vi "TxPkt - Export Channel Configuration.vi"(8 "error in (no error)":errorcluster, 11 "Packet Ref in":T1 format="%.0x") -> (0 "error out":errorcluster, 3 "Packet Ref out":T1 format="%.0x")   [LabVIEW 2019, in "UDP-Custom-Device System Explorer.lvlib"]
uses:
  UDP-Custom-Device System Explorer.lvlib
  <vilib>/NI VeriStand/Custom Device API/Custom Device Item Ref.ctl
  Types/Channel Configuration/Channel Config File Data.ctl
  Property Accessors/Tx Packet Accessors.lvlib
  Property Accessors/Shared Packet Accessors.lvlib
  <vilib>/NI VeriStand/Custom Device API/Custom Device API.lvlib
  Shared/UDP-Custom-Device Shared.lvlib
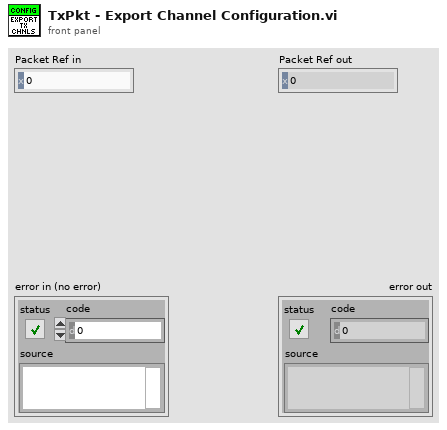
[diagram p1: front panel]
types:
  T1 = typedef "Custom Device API.lvlib/Custom Device Item Ref.ctl" = u64
  T2 = typedef "UDP-Custom-Device System Explorer.lvlib/Channel Config File Data.ctl" = cluster{"Signal Names":string[], "Channel Names":string[], "Channel Data Types":string[], "Channel Descriptions":string[]}
  T3 = typedef "UDP-Custom-Device Shared.lvlib/Shared - Channel Data Type.ctl" = enum16{"Boolean", "Single", "Double", "I8", "I16", "I32", "I64", "U8", "U16", "U32", "U64"}
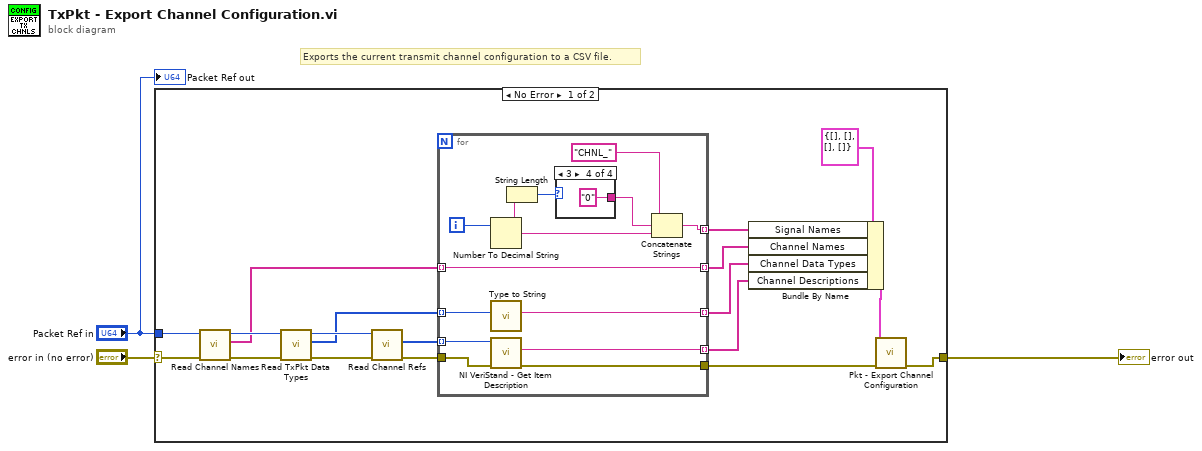
[diagram p0: block diagram]
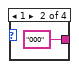
[diagram p3: hidden frame]
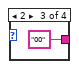
[diagram p4: hidden frame]
diagram:
  # "Exports the current transmit channel configuration to a CSV file."
  n1 = case shown="No Error" "error in (no error)" {
    selector: "error in (no error)" -> [w20 w38]
    tunnel: "Packet Ref in" -> [w21 _]
    tunnel: [w10 w38] -> w2
    frame No Error {
      n2 = call "Read Channel Names.vi"("error in (no error)"=w20, "Node Ptr"=w21) -> ("error out"=w18:errorcluster, "Channel Names"=w12:string[], "Node Ptr out"=w19:T1)  [unwired: 7 in]
      n3 = call "Read TxPkt Data Types.vi"("error in (no error)"=w18, "Node Ptr"=w19) -> ("error out"=w16:errorcluster, "Data types"=w13:T3[], "Node Ptr out"=w17:T1)  [unwired: 7 in]
      n4 = call "Read Channel Refs.vi"("error in (no error)"=w16, "Node Ptr"=w17) -> ("error out"=w15:errorcluster, "Dependent Node Refs"=w14:T1[])  [unwired: 7 in, 1 out]
      n5 = for {
        tunnel: w15 -> [w33]
        tunnel: w14 -> [w34] mode=indexing
        tunnel: [w32] -> w5 mode=indexing
        tunnel: [w31] -> w11
        tunnel: w13 -> [w28] mode=indexing
        tunnel: [w27] -> w6 mode=indexing
        tunnel: [w25] -> w8 mode=indexing
        tunnel: w12 -> [w26] mode=indexing
        tunnel: [w26] -> w7 mode=indexing
        i -> [w30]
        n6 = Number To Decimal String(number=w30) -> (decimal integer string=w24:string)  [unwired: 1 in]
        n7 = call "Type to String.vi"("Data Type"=w28) -> ("String Type"=w27:string)  [unwired: 10 in]
        n8 = call <vilib>:"NI VeriStand - Get Item Description.vi"("error in (no error)"=w33, "Item Ref in"=w34) -> ("error out"=w31:errorcluster, "Description"=w32:string)  [unwired: 6 in, 2 out]
        n9 = String Length(string=w24) -> (length=w23:i32)
        n10 = case shown="3" w23 {
          tunnel: [_ "000" ("Description") "00" ("Description") "0" ("Description")] -> w22
          frame Default {
          }
          frame 1 {
          }
          frame 2 {
          }
          frame 3 {
          }
        }
        n11 = Concatenate Strings("CHNL_" ("Description"), w22, w24) -> (w25:string)
      }
      n12 = Bundle By Name(cluster=T2 {"Signal Names"=[], "Channel Names"=[], "Channel Data Types"=[], "Channel Descriptions"=[]} ("Channel Config Data"), "Signal Names"=w8, "Channel Names"=w7, "Channel Data Types"=w6, "Channel Descriptions"=w5) -> (w4:T2)
      n13 = call "Pkt - Export Channel Configuration.vi"("error in (no error)"=w11, "Channel Config Data"=w4) -> ("error out"=w10:errorcluster)  [unwired: 9 in]
    }
    frame Error {
    }
  }
  "error out" <- w2
  "Packet Ref out" <- "Packet Ref in"
